vi "_Counter.vi"(0 "Dwell (uS)":u32) -> ()   [LabVIEW 2012]
doc: "This VI runs on the FPGA device. It contains a software controlled up / down counter. The direction control sets the direction the counter will count on a rising edge of the source signal. To reset the count value, click the reset button.\n\nMake sure your signal input terminals match the terminal selected under the General Configuration tab of the Configure Digital Input dialog box. Refer to your hardware documentation for information about specific pin numbers.\n\nFPGA Utilization:~ 2%"
uses:
  <vilib>/platform/TimedLoop/XDataNode/XDataNode.xnode
  <vilib>/Platform/TimedLoop/XDataNode/nitl_modes.ctl
  <vilib>/Platform/TimedLoop/XDataNode/XDNodeRunTimeDep.lvlib
  <vilib>/Platform/TimedLoop/XDataNode/wakeup.ctl
  <vilib>/Platform/TimedLoop/XDataNode/timing_clust.ctl
  <vilib>/eio/EIONode/EIONode.xnode
  Instance           1 16Saved   _Counter .vi
  Instance           2 16Saved   _Counter .vi
  <vilib>/rvi/DataTransferAndStorage/Container/XNode/niFpgaContainer.xnode
  <vilib>/rvi/interface/RandomDataEmulation/nirviRandomDataFpgaReadWriteTemplate.vi
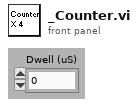
[diagram p1: front panel]
types:
  T1 = typedef "XDNodeRunTimeDep.lvlib/timing_clust.ctl" = cluster{"Expected End [f-1]":u64, "Actual End [f-1]":u64, "Finished Late? [f-1]":bool, "Expected End [i-1]":u64, "Actual End [i-1]":u64, "Finished Late? [i-1]":bool, "Expected Start [i]":u64, "Actual Start [i]":u64, "Expected Start [f]":u64, "Actual Start [f]":u64, "Source Name":string, "Structure Name":string, "Period":i64, "Deadline":i64, "Offset":i64, "Start":i64, "Priority":i32, "Timeout":i32, "Mode":T2, "Wakeup Reason":T3, "Error":errorcluster, "Source Type":string, "Secondary Source Type":string, "Global End Time":u64, "Global Start Time":u64, "Frame Duration":u64, "Iteration Duration":u64, "Assigned CPU":i32, "I/O Scan Engine Mode":u32}
  T2 = typedef "XDNodeRunTimeDep.lvlib/nitl_modes.ctl" = enum32{"No Change", "Process missed periods, maintain original phase", "Discard missed periods, maintain original phase", "Process missed periods, ignore original phase", "Discard missed periods, ignore original phase"}
  T3 = typedef "XDNodeRunTimeDep.lvlib/wakeup.ctl" = enum32{"Normal", "Aborted", "Asynchronous wakeup", "Timing source error", "Timed loop error", "Timeout"}
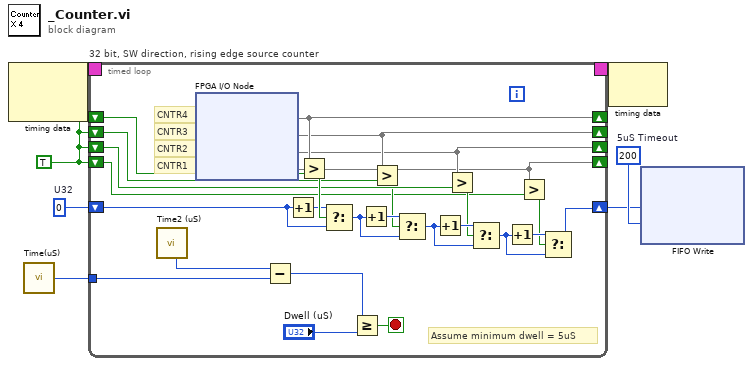
[diagram p0: block diagram]
diagram:
  w7 = u16 200  # 5uS Timeout
  w1 = TRUE ("DIOInput")
  w5 = u32 0  # U32
  n1 = node-c288() -> (w2:T1)  [unwired: 2 out]
  n2 = call "Time(uS)"() -> ("Tick Count(uSec)"=w4:u32)
  n3 = timed-loop "32 bit, SW direction, rising edge source counter" {
    tunnel: w4 -> [w10]
    shift-left: w1 -> [w19]
    shift-right: [w13] -> _
    shift-left: w1 -> [w29]
    shift-right: [w14] -> _
    shift-left: w1 -> [w30]
    shift-right: [w15] -> _
    timing-out: [_] -> w3
    timing: w2 -> [_]
    shift-left: w5 -> [w31]
    shift-right: [w17] -> w6
    shift-left: w1 -> [w22]
    shift-right: [w16] -> _
    stop <- w11 stop-if-true
    # "CNTR1"
    # "CNTR2"
    # "CNTR3"
    # "CNTR4"
    # "Assume minimum dwell = 5uS"
    n4 = call "Time2 (uS)"() -> ("Tick Count(uSec)"=w9:u32)
    n5 = xnode "FPGA I/O Node"() -> ("Port0/DIO0"=w16, "Port0/DIO1"=w15, "Port0/DIO2"=w14, "Port0/DIO3"=w13)  [unwired: 4 in, 4 out]
    n6 = Subtract(x=w9, y=w10) -> (x-y=w8:u32)
    n7 = Increment(x=w31) -> (x+1=w32:u32)
    n8 = Greater?(x=w16, y=w22) -> (0:w33:bool)
    n9 = Select(t=w32, s=w33, f=w31) -> (s? t:f=w26:u32)
    n10 = Greater Or Equal?(x=w8, y="Dwell (uS)") -> (x >= y?=w11:bool)
    n11 = Increment(x=w26) -> (x+1=w28:u32)
    n12 = Greater?(x=w15, y=w30) -> (0:w27:bool)
    n13 = Select(t=w28, s=w27, f=w26) -> (s? t:f=w24:u32)
    n14 = Increment(x=w24) -> (x+1=w25:u32)
    n15 = Greater?(x=w14, y=w29) -> (0:w23:bool)
    n16 = Select(t=w25, s=w23, f=w24) -> (s? t:f=w20:u32)
    n17 = Increment(x=w20) -> (x+1=w21:u32)
    n18 = Greater?(x=w13, y=w19) -> (0:w18:bool)
    n19 = Select(t=w21, s=w18, f=w20) -> (s? t:f=w17:u32)
  }
  n20 = node-c288(w3) -> ()  [unwired: 1 out]
  n21 = xnode ("FIFO Write")("Element"=w6, "Timeout"=w7) -> ()  [unwired: 1 in, 2 out]
